vi "DecodeRecord.vi"(11 "wpilog (bytes)":u8[](array[numeric]) format="%x") -> (1 "record":T1, 3 "rest of the log":u8[](array[numeric]))   [LabVIEW 2023]
panel:
  out "timestamp microSec":i32
  out "payload size":i32
  out "entry ID":i32
  out "payload size length  (bytes)":u32
  out "ID length (bytes)":u32
  out "timestamp length (bytes)":u32
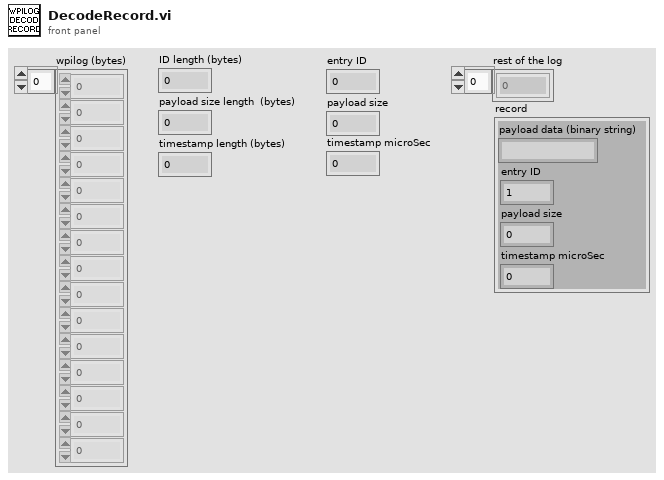
[diagram p1: front panel]
types:
  T1 = cluster{"payload data (binary string)":string, "entry ID":i32, "payload size":i32, "timestamp microSec":i32}
  T2 = enum16{"big-endian, network order", "native, host order", "little-endian"}
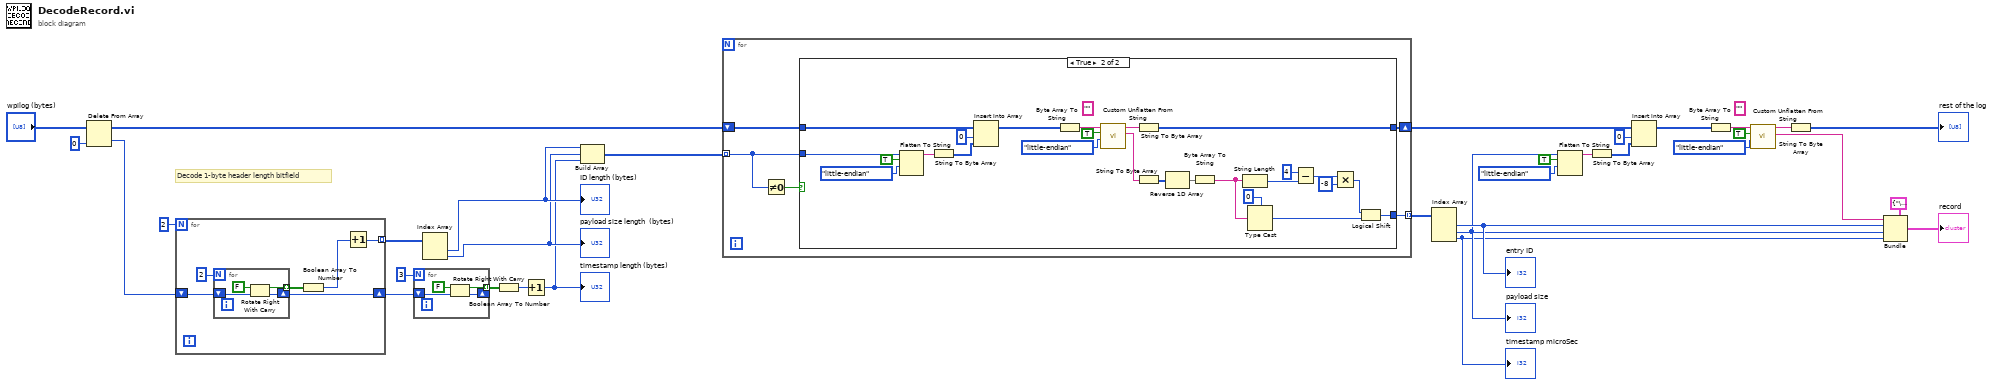
[diagram p0: block diagram]
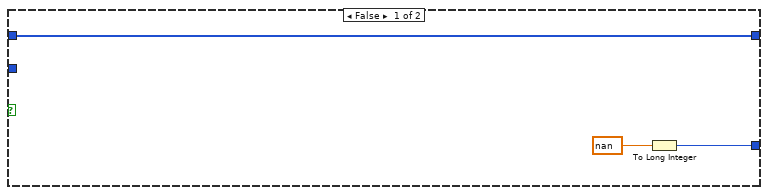
[diagram p2: hidden frame]
diagram:
  (unwired) ""
  # "Decode 1-byte header length bitfield"
  n1 = Delete From Array(array="wpilog (bytes)", index=0) -> (deleted portion=w25:u8, array with subset deleted=w20:u8[])  [unwired: 1 in]
  n2 = for {
    N: 2 -> [_]
    shift-right: [w37] -> w31
    shift-left: w25 -> [w36]
    tunnel: [w34] -> w28 mode=indexing
    n3 = for {
      N: 2 -> [_]
      shift-right: [w41] -> w37
      shift-left: w36 -> [w43]
      tunnel: [w40] -> w38 mode=indexing
      n4 = Rotate Right With Carry(2:w43, 3:FALSE ("carry")) -> (0:w41:u8, 1:w40:bool)
    }
    n5 = Boolean Array To Number(Boolean array=w38) -> (number=w35:u32)
    n6 = Increment(x=w35) -> (x+1=w34:u32)
  }
  n7 = for {
    N: 3 -> [_]
    shift-right: [w45] -> _
    shift-left: w31 -> [w47]
    tunnel: [w44] -> w30 mode=indexing
    n8 = Rotate Right With Carry(2:w47, 3:FALSE ("carry")) -> (0:w45:u8, 1:w44:bool)
  }
  n9 = Index Array(array=w28) -> (element #1=w24:u32, element #2=w23:u32)  [unwired: 2 in]
  "ID length (bytes)" <- w24
  "payload size length  (bytes)" <- w23
  n10 = Boolean Array To Number(Boolean array=w30) -> (number=w29:u32)
  n11 = Increment(x=w29) -> (x+1=w22:u32)
  "timestamp length (bytes)" <- w22
  n12 = Build Array(w24, w23, w22) -> (w21:u32[])
  n13 = for {
    tunnel: w21 -> [w49] mode=indexing
    shift-right: [w52] -> w13
    shift-left: w20 -> [w51]
    tunnel: [w50] -> w19 mode=indexing
    n14 = Not Equal To 0?(x=w49) -> (x != 0?=w48:bool)
    n15 = case shown="True" w48 {
      tunnel: [w55 w74] -> w52
      tunnel: w51 -> [w55 w73]
      tunnel: w49 -> [_ w72]
      tunnel: [w53 w61] -> w50
      frame False {
        n16 = To Long Integer(number=nan) -> (32bit integer=w53:i32)
      }
      frame True {
        (unwired) ""
        n17 = Flatten To String(anything=w72, prepend array or string size? (T)=TRUE, byte order (0:big-endian, network order)=T2."little-endian") -> (data string=w78:string)  [unwired: 1 in, 2 out]
        n18 = String To Byte Array(string=w78) -> (unsigned byte array=w76:u8[])
        n19 = Insert Into Array(array=w73, index=0, new element=w76) -> (w75:u8[])
        n20 = Byte Array To String(unsigned byte array=w75) -> (string=w60:string)
        n21 = call "Custom Unflatten From String.vi"("byte order (0:big-endian, network order)"=T2."little-endian", "data includes array or string size? (T)"=TRUE, "binary string"=w60) -> ("value"=w58:string, "rest of the binary string"=w59:string)  [unwired: 7 in]
        n22 = String To Byte Array(string=w59) -> (unsigned byte array=w74:u8[])
        n23 = String To Byte Array(string=w58) -> (unsigned byte array=w71:u8[])
        n24 = Reverse 1D Array(array=w71) -> (reversed array=w70:u8[])
        n25 = Byte Array To String(unsigned byte array=w70) -> (string=w62:string)
        n26 = String Length(string=w62) -> (length=w66:i32)
        n27 = Type Cast(type=0, x=w62) -> (*(type *) &x=w68:i32)
        n28 = Subtract(x=4, y=w66) -> (x-y=w67:i32)
        n29 = Multiply(x=w67, y=-8) -> (x*y=w64:i32)
        n30 = Logical Shift(y=w64, x=w68) -> (x << y=w61:i32)
      }
    }
  }
  n31 = Index Array(array=w19) -> (element #1=w10:i32, element #2=w9:i32, element #3=w8:i32)  [unwired: 3 in]
  "entry ID" <- w10
  "payload size" <- w9
  "timestamp microSec" <- w8
  n32 = Flatten To String(anything=w9, prepend array or string size? (T)=TRUE, byte order (0:big-endian, network order)=T2."little-endian") -> (data string=w16:string)  [unwired: 1 in, 2 out]
  n33 = String To Byte Array(string=w16) -> (unsigned byte array=w14:u8[])
  n34 = Insert Into Array(array=w13, index=0, new element=w14) -> (w12:u8[])
  n35 = Byte Array To String(unsigned byte array=w12) -> (string=w3:string)
  n36 = call "Custom Unflatten From String.vi"("byte order (0:big-endian, network order)"=T2."little-endian", "data includes array or string size? (T)"=TRUE, "binary string"=w3) -> ("value"=w5:string, "rest of the binary string"=w4:string)  [unwired: 7 in]
  n37 = String To Byte Array(string=w4) -> (unsigned byte array=→"rest of the log":u8[])
  n38 = Bundle(cluster=T1 {"payload data (binary string)"="\u0000\u0000\u0000\u0000\u0000\u0000\u0000\u0003", "entry ID"=1, "payload size"=0, "timestamp microSec"=0} ("record"), "payload data (binary string)"=w5, "entry ID"=w10, "payload size"=w9, "timestamp microSec"=w8) -> (→"record":T1)
